vi "AlliGator Get Phasor Plot Parameters.vi"(8 "Error In":errorcluster) -> (0 "Error Out":errorcluster, 3 "Phasor Plot Parameters":T1={"Phasor Frequency"=0.0, "Decay Preprocessing Options & Parameters"={"Background Subtraction Parameters"={"Background Definition Range"={"Min Gate"=0.0, "Max Gate"=0.0}, "Baseline Subtraction Method"=enum."Mean", "Background Subtraction?"=FALSE, "Background File"=path "", "Background Constant"=0.0, "Background Scaling Factor"=1.0, "Background Pile-up Correction"=FALSE, "Background Pixel Well Capacity"=1}, "Decay Preprocessing Parameters"={"Background Subtraction"=FALSE, "Straighten Decay"=FALSE, "Reverse Gates"=FALSE, "1-Normalized Decay"=FALSE, "Smoothen Decay"=FALSE, "Smoothing Parameter"=0.0, "Shift Decay"=FALSE, "Decay Shift Parameters"={"Type"=enum."Default", "Shift"=0.0, "Threshold"=0.0, "Rotate"=FALSE}, "Extrapolate Decay"=FALSE, "Additional Points"=0, "Head Fraction"=0.0, "Pixel-Normalize Decay"=FALSE, "Use Periodicity"=FALSE, "Use Cursors"=FALSE, "Tail Fraction"=0.0, "Use Decay Pre-Processing"=TRUE, "Fold Decay"=FALSE, "# Folds"=1, "[0-1]-Normalized Decay"=FALSE}, "Preprocessing Steps Order"=[]}, "FLI Dataset Modified"=FALSE, "Source Image Settings"={"Low Count Pixels Rejection Options"={"Background Low Threshold Factor"=0.0, "Fixed Low Background Threshold"=0.0, "Reject Low Count Pixels"=FALSE, "Low Percentile"=0.0}, "High Count Pixels Rejection Options"={"Background High Threshold Factor"=0.0, "Fixed High Background Threshold"=20000.0, "Reject High Count Pixels"=FALSE, "High Percentile"=100.0}}, "Data Information"={"Gate Width"=0.0, "Gate Separation"=0.0, "Step (Gate Separation)"=0, "Laser Period"=0.0, "SYNC Period"=0.0, "Channel Name"=0, "Channel Arithmetic"=enum."None", "Pile-up Correction"=FALSE, "Pixel Well Capacity"=1, "Dataset Scaling Factor"=1.0}, "Phasor Plot"={"Phasor Plot Smoothing Options"={"Use Phasor Plot Smoothing"=FALSE, "Kernel Type"=enum."Uniform", "Bin"=1, "Algorithm"=enum."Rapid"}, "Phasor Plot Size"={"H"=0, "V"=0, "Margin"=0.0}, "Selected Image ROI(s)"=FALSE, "All Image ROIs"=FALSE, "Selected Source Image ROI"=0, "Source Image ROIs"=[]}} {"Phasor Plot"."Source Image ROIs"."ROI Descriptor"."Contours"."Type" items=["No Selection", "Point", "Line", "Rectangle", "Oval", "Polygon", "Freehand Region", "Annulus", "Unused2", "Unused3", "Broken Line", "Freehand Line", "Rotated Rectangle"]; "Phasor Plot"."Phasor Plot Smoothing Options"."Bin" min=1 step=2; "Data Information"."Dataset Scaling Factor" min=0.0; "Data Information"."Pixel Well Capacity" min=1 step=1; "Data Information"."Channel Name" items=["Gate"]; "Source Image Settings"."High Count Pixels Rejection Options"."High Percentile" min=0.0 max=100.0; "Source Image Settings"."Low Count Pixels Rejection Options"."Low Percentile" min=0.0 max=100.0; "Decay Preprocessing Options & Parameters"."Decay Preprocessing Parameters"."# Folds" min=1; "Decay Preprocessing Options & Parameters"."Background Subtraction Parameters"."Background Pixel Well Capacity" min=1 step=1; "Phasor Frequency" min=-2147483648.0 max=2147483647.0}, 4 "CPU (s)":dbl)   [LabVIEW 2021, in "AlliGator Phasor Plot.lvlib"]
doc: "Returns a structure with all the options needed to build the Phasor Plot image."
uses:
  AlliGator Phasor Plot.lvlib
  AlliGator Phasor Plot Parameters v2.ctl
  Decay Analysis/Decay Preprocessing/AlliGator Decay Preprocessing Options.ctl
  Decay Analysis/Decay Preprocessing/AlliGator Background Subtraction Parameters.ctl
  Decay Analysis/Decay Preprocessing/AlliGator Baseline Subtraction Method.ctl
  Decay Analysis/Decay Preprocessing/AlliGator Decay Preprocessing Parameters.ctl
  Graphs/XY Graph/XY Graph Plot Shift Parameters.ctl
  Graphs/XY Graph/XY Graph Plot Shift Method.ctl
  Settings/AlliGator Low Count Pixels Rejection Options.ctl
  Settings/AlliGator High Count Pixels Rejection Options.ctl
  Settings/AlliGator Gate Arithmetic.ctl
  AlliGator Phasor Plot Smoothing Options.ctl
  Arrays/Kernel Type.ctl
  Arrays/Smoothing Algorithm.ctl
  AlliGator Phasor Plot Size.ctl
  Image/Named ROI Description.ctl
  Settings/AlliGator Settings List.ctl
  Globals, Variables, Constants/AlliGator Variables List.ctl
  Variant/Variant to Data/Variant to I32.vi
  Variant/Variant to Data/Variant to Boolean.vi
  Settings/AlliGator Settings.lvlib
  Arrays/Arrays.lvlib
  Variant/Variant to Data/Variant to Data.lvlib
  Graphs/XY Graph/XY Graph Add-Ons.lvlib
  Decay Analysis/Decay Preprocessing/AlliGator Decay Preprocessing.lvlib
  Globals, Variables, Constants/AlliGator Globals, Variables & Constants.lvlib
  Image/Image.lvlib
  Time/Time.lvlib
panel:
  # "see the AlliGator License on the block diagram (Ctrl+E or Window:Show Block Diagram)"
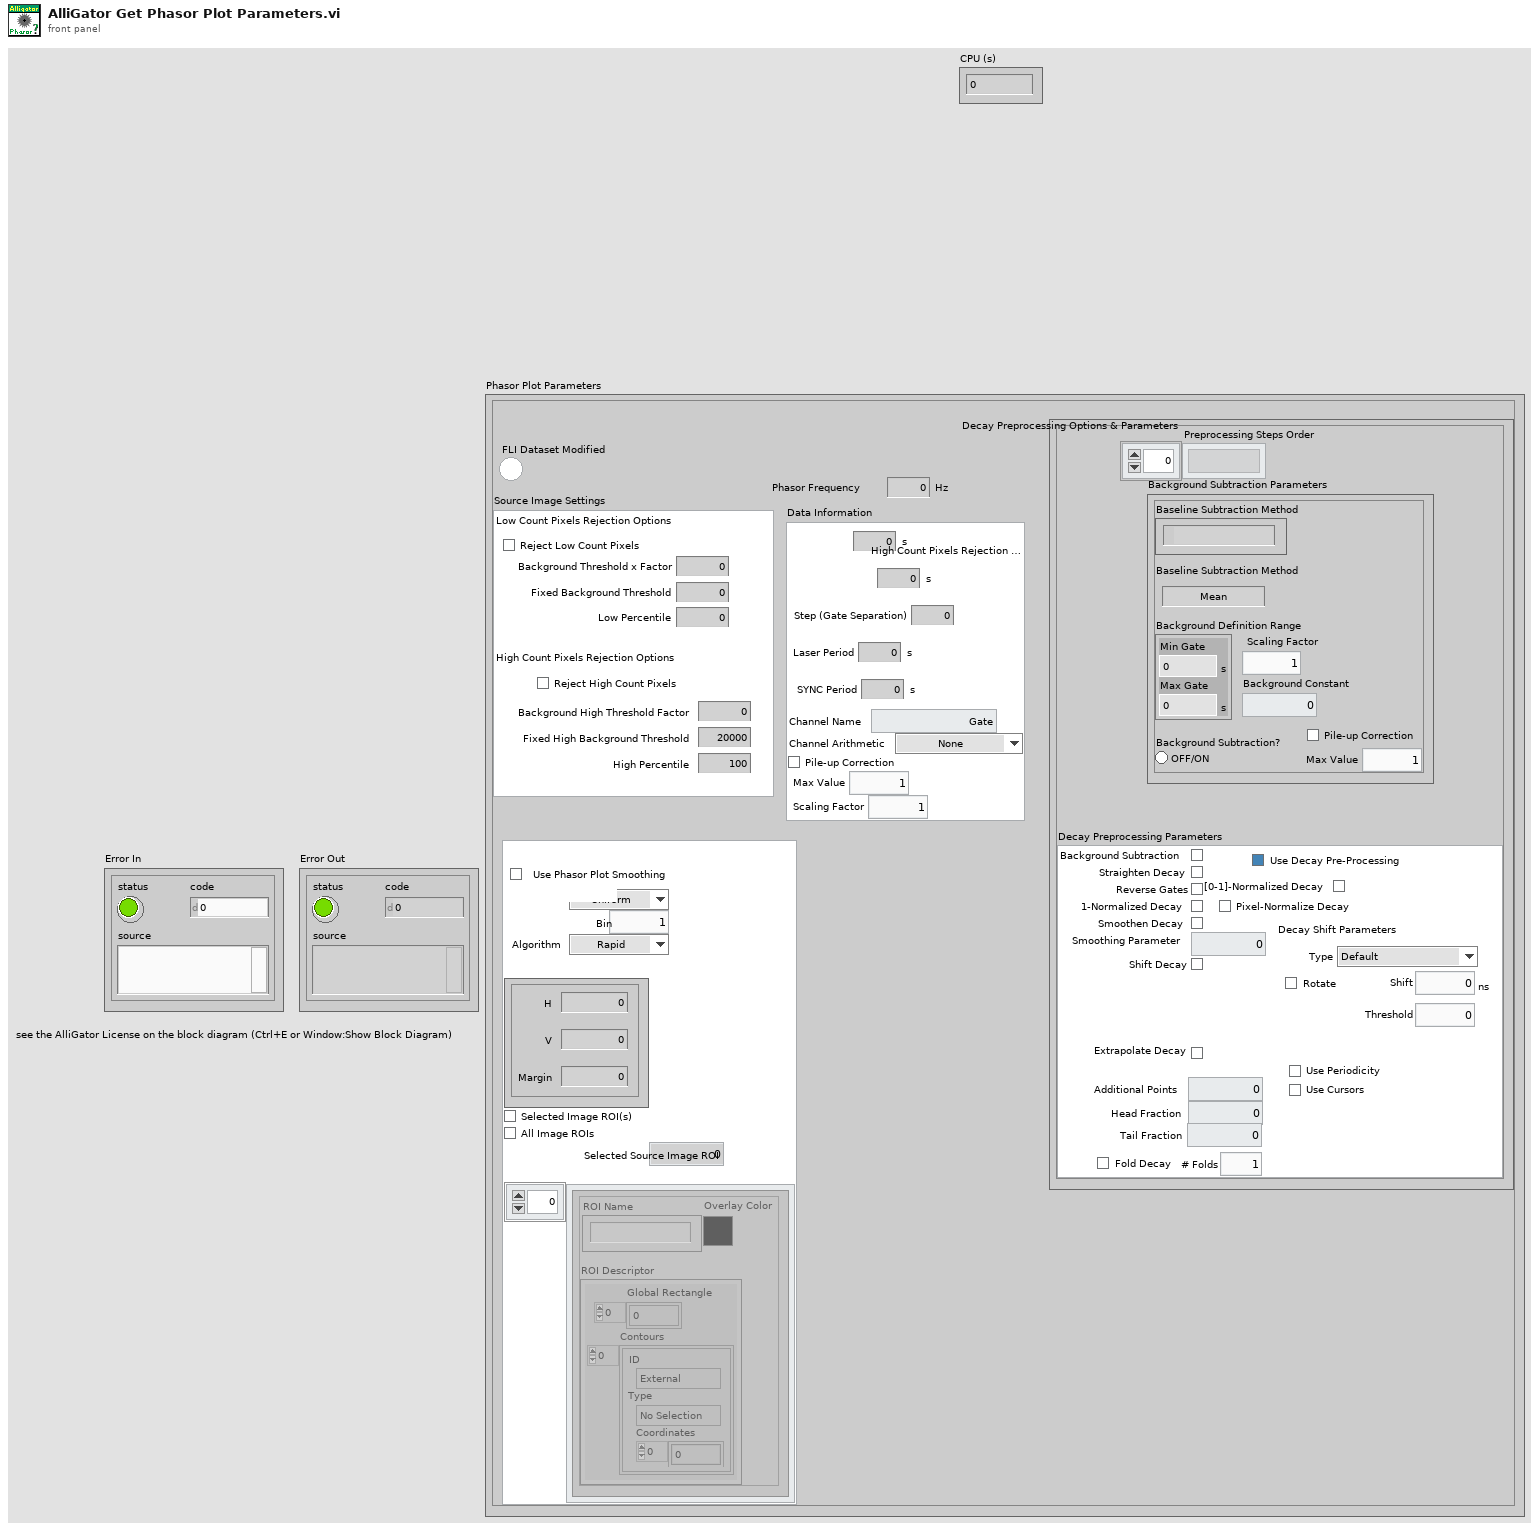
[diagram p1: front panel]
types:
  T1 = typedef "AlliGator Phasor Plot.lvlib/AlliGator Phasor Plot Parameters v2.ctl" = cluster{"Phasor Frequency":dbl[unit], "Decay Preprocessing Options & Parameters":T2, "FLI Dataset Modified":bool, "Source Image Settings":cluster{"Low Count Pixels Rejection Options":T8, "High Count Pixels Rejection Options":T9}, "Data Information":cluster{"Gate Width":dbl[unit], "Gate Separation":dbl[unit], "Step (Gate Separation)":i32, "Laser Period":dbl[unit], "SYNC Period":dbl[unit], "Channel Name":u16, "Channel Arithmetic":T10, "Pile-up Correction":bool, "Pixel Well Capacity":u32, "Dataset Scaling Factor":dbl}, "Phasor Plot":cluster{"Phasor Plot Smoothing Options":T11, "Phasor Plot Size":T14, "Selected Image ROI(s)":bool, "All Image ROIs":bool, "Selected Source Image ROI":i32, "Source Image ROIs":T15[]}}
  T2 = typedef "AlliGator Decay Preprocessing.lvlib/AlliGator Decay Preprocessing Options.ctl" = cluster{"Background Subtraction Parameters":T3, "Decay Preprocessing Parameters":T5, "Preprocessing Steps Order":string[]}
  T3 = typedef "AlliGator Decay Preprocessing.lvlib/AlliGator Background Subtraction Parameters.ctl" = cluster{"Background Definition Range":cluster{"Min Gate":dbl[unit], "Max Gate":dbl[unit]}, "Baseline Subtraction Method":T4, "Background Subtraction?":bool, "Background File":path, "Background Constant":dbl, "Background Scaling Factor":dbl, "Background Pile-up Correction":bool, "Background Pixel Well Capacity":u32}
  T4 = typedef "AlliGator Decay Preprocessing.lvlib/AlliGator Baseline Subtraction Method.ctl" = enum16{"Mean", "Min", "Square Gated Single-Exponential", "File", "Constant"}
  T5 = typedef "AlliGator Decay Preprocessing.lvlib/AlliGator Decay Preprocessing Parameters.ctl" = cluster{"Background Subtraction":bool, "Straighten Decay":bool, "Reverse Gates":bool, "1-Normalized Decay":bool, "Smoothen Decay":bool, "Smoothing Parameter":dbl, "Shift Decay":bool, "Decay Shift Parameters":T6, "Extrapolate Decay":bool, "Additional Points":u32, "Head Fraction":dbl, "Pixel-Normalize Decay":bool, "Use Periodicity":bool, "Use Cursors":bool, "Tail Fraction":dbl, "Use Decay Pre-Processing":bool, "Fold Decay":bool, "# Folds":u32, "[0-1]-Normalized Decay":bool}
  T6 = typedef "XY Graph Add-Ons.lvlib/XY Graph Plot Shift Parameters.ctl" = cluster{"Type":T7, "Shift":dbl[unit], "Threshold":dbl, "Rotate":bool}
  T7 = typedef "XY Graph Add-Ons.lvlib/XY Graph Plot Shift Method.ctl" = enum16{"Default", "CFD", "Threshold", "Cross-Correlation"}
  T8 = typedef "AlliGator Settings.lvlib/AlliGator Low Count Pixels Rejection Options.ctl" = cluster{"Background Low Threshold Factor":dbl, "Fixed Low Background Threshold":dbl, "Reject Low Count Pixels":bool, "Low Percentile":dbl}
  T9 = typedef "AlliGator Settings.lvlib/AlliGator High Count Pixels Rejection Options.ctl" = cluster{"Background High Threshold Factor":dbl, "Fixed High Background Threshold":dbl, "Reject High Count Pixels":bool, "High Percentile":dbl}
  T10 = typedef "AlliGator Settings.lvlib/AlliGator Gate Arithmetic.ctl" = enum16{"None", "INT-G2", "G2/INT*<INT>", "(1 - G2/INT)*<INT>"}
  T11 = typedef "AlliGator Phasor Plot.lvlib/AlliGator Phasor Plot Smoothing Options.ctl" = cluster{"Use Phasor Plot Smoothing":bool, "Kernel Type":T12, "Bin":i32, "Algorithm":T13}
  T12 = typedef "Arrays.lvlib/Kernel Type.ctl" = enum16{"Uniform", "Bilinear", "Gaussian"}
  T13 = typedef "Arrays.lvlib/Smoothing Algorithm.ctl" = enum16{"Rapid", "Thorough"}
  T14 = typedef "AlliGator Phasor Plot.lvlib/AlliGator Phasor Plot Size.ctl" = cluster{"H":i32, "V":i32, "Margin":dbl}
  T15 = typedef "Image.lvlib/Named ROI Description.ctl" = cluster{"ROI Descriptor":T16, "ROI Name":string, "Overlay Color":u32}
  T16 = typedef "ROI Descriptor" = cluster{"Global Rectangle":i32[], "Contours":cluster{"ID":enum32{"External", "Internal"}, "Type":u32, "Coordinates":i32[]}[]}
  T17 = typedef "AlliGator Settings.lvlib/AlliGator Settings List.ctl" = enum16{"GUI:Visible Settings Tab", "GUI:Last Run Version", "Source Image:Use Image Histogram for Contrast", "Source Image:Low Count Pixels Rejection Options", "Source Image:High Count Pixels Rejection Options", "Source Image:Use Image Brightness", "Source Image:Blend Overlay with Image Background", "Source Image:Use Fixed ROI Diameter", "Source Image:ROI Diameter", "Source Image:ROI Center Color", "Source Image:Peak Threshold", "Source Image:Intensity Threshold", "Source Image:Image Binning Options", "Source Image:Image Smoothing Options", "Source Image:Image Histogram Active", "Source Image:Invert Binary Mask", "Source Image:Hot Pixel Removal", "Source Image:Overlay Analyzed ROI Center", "Source Image:Auto-Adjust Contrast", "Source Image:Histogram Lower Percentile", "Source Image:Histogram Upper Percentile", "Source Image:Save Source Image", "Source Image:Scale Bar Options", "Source Image:Image Resolution (Pixel Size)", "Source Image:Flatfield Correction", "Source Image:Show Dead Left Columns Correction", "Source Image:Dead Left Columns Correction", "Source Image:Image Pre-Processing Operations Order", "Source Image:Overlay ROI Median", "Source Image:Median Overlay Color", "Data Information:Gate Width", "Data Information:Nanotime Gate Separation", "Data Information:Macrotime Gate Separation", "Data Information:Gate Step", "Data Information:# Gates", "Data Information:Gate Image Exposure", "Data Information:Gate Image Integration", "Data Information:Gates to Skip", "Data Information:Gates to Keep", "Data Information:Define Gates to", "Data Information:Channel Name", "Data Information:Available Channel Names", "Data Information:Channel Arithmetic", "Data Information:Background File Subtraction", "Data Information:Background File", "Data Information:Background Scaling Factor", "Data Information:Background Pile-up Correction", "Data Information:Background Pixel Well Capacity", "Data Information:Laser Period", "Data Information:SYNC Period", "Data Information:Pile-up Correction", "Data Information:Pixel Well Capacity", "Data Information:Dataset Scaling Factor", "Fluorescence Decay_Decay Pre-Processing:Reverse Gates", "Fluorescence Decay_Decay Pre-Processing:Verbose Decay Pre-Processing", "Fluorescence Decay_Decay Pre-Processing:Use Decay Pre-Processing", "Fluorescence Decay_Decay Pre-Processing:Background Subtraction", "Fluorescence Decay_Decay Pre-Processing:Background Definition Range", "Fluorescence Decay_Decay Pre-Processing:Baseline Subtraction Method", "Fluorescence Decay_Decay Pre-Processing:Decay Pre-Processing Operations Order", "Fluorescence Decay_Decay Pre-Processing:Smoothing Parameter", "Fluorescence Decay_Decay Pre-Processing:Shift Decay", "Fluorescence Decay_Decay Pre-Processing:Decay Shift Parameters", "Fluorescence Decay_Decay Pre-Processing:Fold Decay", "Fluorescence Decay_Decay Pre-Processing:# Folds", "Fluorescence Decay_Decay Pre-Processing:1-Normalize Decay", "Fluorescence Decay_Decay Pre-Processing:[0-1]-Normalize Decay", "Fluorescence Decay_Decay Pre-Processing:Smoothen Decay", "Fluorescence Decay_Decay Pre-Processing:Extrapolate Decay", "Fluorescence Decay_Decay Pre-Processing:Use Periodicity", "Fluorescence Decay_Decay Pre-Processing:Use Cursors", "Fluorescence Decay_Decay Pre-Processing:Tail Fraction", "Fluorescence Decay_Decay Pre-Processing:Head Fraction", "Fluorescence Decay_Decay Pre-Processing:Additional Points", "Fluorescence Decay_Decay Pre-Processing:Straighten Decay", "Fluorescence Decay_Decay Pre-Processing:Constant Background", "Fluorescence Decay_Decay Pre-Processing:Pixel-Normalize Decay", "Fluorescence Decay_Advanced Analysis:Extract IRF instead of Decay", "Fluorescence Decay_Advanced Analysis:IRF Extraction Options", "Fluorescence Decay_Advanced Analysis:IRF Optimization Options", "Fluorescence Decay_Advanced Analysis:Square Pulse Options", "Fluorescence Decay_Advanced Analysis:IRF Order", "Fluorescence Decay_Advanced Analysis:IRF Time Constants", "Fluorescence Decay_Advanced Analysis:Wavelet Analysis Options", "Fluorescence Decay_Advanced Analysis:Average Lifetime Options", "Fluorescence Decay_Fit Options:Fit Options", "Fluorescence Decay_Fit Options:Use Legacy Fitting Approach", "Fluorescence Decay_Fit Options:Use Data Information Laser Period", "Fluorescence Decay_Fit Parameters:Displayed Fit Parameters", "Fluorescence Decay_Fit Parameters:Fit Parameter Constraints", "Fluorescence Decay_Fit Parameters:Export Tabulated Results", "Fluorescence Decay_Fit Parameters:MLE Baseline Offset Type", "Fluorescence Decay_Fit Parameters:MLE Baseline Offset", "Fluorescence Decay_Fit Parameters:Guess Parameter Names", "Fluorescence Decay_Fit Parameters:Guess Parameter Values", "Fluorescence Decay_Fit Parameters:Guess Parameters Options", "Fluorescence Decay_Styles:Show Last Decay Only", "Fluorescence Decay_Styles:Decay Graph Color Array", "Fluorescence Decay:Decay Graph Active", "Fluorescence Decay Statistics:Min Peak Value", "Fluorescence Decay Statistics:Reject Low Decay Peak Pixels", "Fluorescence Decay Statistics:Reject High Decay Peak Pixels", "Fluorescence Decay Statistics:Max Peak Value", "Time Traces:Use File Timestamp", "Time Traces:Time Step", "Time Traces:Use Intensity Correction File", "Time Traces:Intensity Correction File", "Phasor Plot:Phasor Plot Smoothing Options", "Phasor Plot:Phasor Plot Size", "Phasor Plot:Phasor Plot Graphics Options", "Phasor Plot:Cumulative Phasor Plot", "Phasor Plot:Use Phasor Brightness", "Phasor Plot:Blend Overlay with Phasor Background", "Phasor Plot:Save Phasor Plot", "Phasor Plot:Show References", "Phasor Plot:Phasor Ratio Decay Range", "Phasor Plot:Exponential Fading", "Phasor Plot:Phasor Ratio Reference Colors", "Phasor Plot:Reference Radius", "Phasor Plot:Show Color Map Vertices", "Phasor Plot:Phasor Plot Active", "Phasor Plot:Phasor Ratio Color Map Type", "Phasor Plot:Phasor Ratio Color Map", "Phasor Plot:Phasor Ratio Display Range", "Phasor Plot:Selected Image ROI(s)", "Phasor Plot:All Image ROIs", "Phasor Plot:Selected Phasor Plot ROI(s)", "Phasor Plot:All Phasor Plot ROIs", "Phasor Plot:Phasor Ratio Color-Coded Quantity", "Phasor Plot:Store Phasor Harmonics", "Phasor Plot:Draw Reference Segment", "Phasor Plot:User-Defined Quantity", "Phasor Graph:Phasor Frequency", "Phasor Graph:Phasor Ratio Type", "Phasor Graph:Pixel-level Phasor Computation", "Phasor Graph:Save Phasor Graph", "Phasor Graph:Phasor Graph Active", "Phasor Graph:Phasor SDV Options", "Phasor Calibration:Use Backup Calibration if needed", "Phasor Graph:Define Shortest Lifetime as", "Phasor Calibration:Backup Calibration Type", "Phasor Calibration:Calibration Type", "Phasor Calibration:Calibration Lifetime", "Phasor Calibration:Calibration Map Algorithm", "Single-Exponential Phasor Locus (SEPL):Gate Parameters", "Single-Exponential Phasor Locus (SEPL):User-defined Gate", "Single-Exponential Phasor Locus (SEPL):User-defined IRF", "Single-Exponential Phasor Locus (SEPL):Phasor Parameters", "Single-Exponential Phasor Locus (SEPL):Decay & IRF Parameters", "Single-Exponential Phasor Locus (SEPL):Display Parameters", "Lifetime Analysis:Decay Analysis Parameters", "Lifetime Analysis:Lifetime Map Active", "Plugins:Python Settings", "Miscellaneous:Verbose Mode", "Miscellaneous:Beep after Script", "Miscellaneous:Saved Image File Format", "Miscellaneous:Exported Gate Image Settings", "Miscellaneous:Include Loading in Timing", "Miscellaneous:Verbose Settings Mode", "Miscellaneous:Histogram Options", "Miscellaneous:Beep on Error", "Miscellaneous:# Logical Processors Used", "Miscellaneous:ROI Description Max Characters", "Miscellaneous:Verbose Error Mode", "Miscellaneous:Transparent Mask Color"}
  T18 = typedef "AlliGator Globals, Variables & Constants.lvlib/AlliGator Variables List.ctl" = enum16{"---- GUI ----", "GUI:Initialization Status", "GUI:State Indicators Refnum", "GUI:Original AlliGator Menu Items", "GUI:Current Action Loop State", "GUI:Script in progress", "GUI:Playback", "GUI:Loop Playback", "GUI:Search ROI Used", "GUI:Search ROI", "Decay Graph Max Legend Size", "Intensity Graph Max Legend Size", "Decay Statistics Graph Max Legend Size", "Phasor Graph Max Legend Size", "Phasor Ratio Graph Max Legend Size", "Lifetime Graph Max Legend Size", "---- Files ----", "Files:Export Dataset Frames as Individual Files", "Files:Show Batch Export Help Balloons", "Files:Frames in Dataset", "Files:ptu File Frame Start Indices", "Files:Current Frame in Dataset", "Files:Current Frame Timestamp", "Files:Dataset Loaded", "Files:Dataset Metadata", "Files:Dataset Channel", "Files:Dataset Data Description", "Files:Background Dataset Metadata", "Files:Background Dataset Channel", "Files:Background Dataset Data Description", "Files:Background File Subtraction", "Files:Background File Path", "Files:Background File Pile-up Correction", "Files:Background File Pixel Well Capacity", "Files:Background File Scaling Factor", "Files:Current Dataset Load Settings", "Files:Dataset Path", "Files:ICCD-specific Information", "Files:Macrotime Gate Separation", "------ Python Plugins ------", "Python Plugins:Information", "Python Plugins:Python Session", "Python Plugins:Valid Python Session?", "---- Source Image ----", "Source Image:ROIs", "Source Image:Current ROI", "Source Image:ROI Event Refnum", "X_Source Image Display Range", "X_Source Image Palette Information", "X_Type of Displayed Image", "X_Time Gate Slider", "Source Image:Palette List", "Source Image:Scale", "Source Image:ROI Overlay Color", "Source Image:Overlay to Erase", "Source Image:Is Displayed Image Accumulated", "Source Image:White Light Image Modified", "Source Image:Mask Image Modified", "---- Image Profile Window ----", "Image Profile:Window Event Refnum", "Image Profile:IntensityType", "Image Profile:Intensity Average Type", "Image Profile:Intensity-weighted SDV", "Image Profile:Box Profile Type", "Image Profile:Window Open", "Image Profile:Plotted Fit Parameter", "------ Phasor Graph -------", "Phasor Graph:Show Line", "---- Phasor Plot ---", "Phasor Plot:Parameters Changed", "Phasor Plot:FLI Dataset Modified since last Calculation", "Phasor Harmonics Data", "Selected Phasor Harmonics", "Phasor Harmonic Manager Event Refnum", "Phasor Plot:ROIs", "Phasor Plot:Current ROI", "Phasor Plot:ROI Event Refnum", "Phasor Plot:Image Reference Points", "Phasor Plot:Computed", "Phasor Plot:Palette Information", "Phasor Plot:Palette List", "Phasor Plot:Phasor Ratio Palette Information", "Phasor Plot:Phasor Ratio Palette List", "Phasor Plot:Image Scale", "Phasor Plot:Image Overlay to Erase", "Phasor Plot:Image Elements to Update", "Phasor Plot:Current Calculation Parameters", "Phasor Plot:Current Calibration Options", "Phasor Plot:Reset Cumulated Phasor Plot", "Phasor Plot:Reference 1", "Phasor Plot:Lifetime Reference 1", "Phasor Plot:Reference 1 Frequency", "Phasor Plot:Reference 2", "Phasor Plot:Lifetime Reference 2", "Phasor Plot:Reference 2 Frequency", "---- Decay Analysis ----", "Number of Selected Decays to Fit", "LS Fit Results", "LAR Fit Results", "BS Fit Results", "Last Decay Max - Min", "Best Fit Parameters", "Best Fit Parameter Names", "Actual Size X", "Actual Size Y", "Binning X", "Binning Y", "Actual # Gates", "Dataset Number", "Gates to...", "Gates Skipped", "Gates to keep", "Gate Step", "Gate Separation", "Reversed Gates", "Pile-up Correction", "Pixel Well Capacity", "Background Subtracted", "Background Subtraction Method", "Background Definition Range", "Background File (deprecated)", "Number of Dataset Accumulated", "Array of Accumulated Dataset Paths", "Do Averaged Datasets", "Destination File Path", "Process Plot Target", "Use 1/D as Phasor Frequency", "---- Decay Fit Parameter Map -----", "Decay Fit Parameter Map:Palette Information", "Decay Fit Parameter Map:Palette List", "---- Parameter Map ----", "Parameter Map:Palette Information", "Parameter Map:Palette List", "------- Local Decay Window ---------", "Local Decay Graph Window:Event Refnum", "Local Decay Graph Window:Use normalized IRF for convolution", "----- Miscellaneous ----", "Misc:Skippable Dialog Windows Status"}
  T19 = cluster{"Min Gate":dbl[unit], "Max Gate":dbl[unit]}
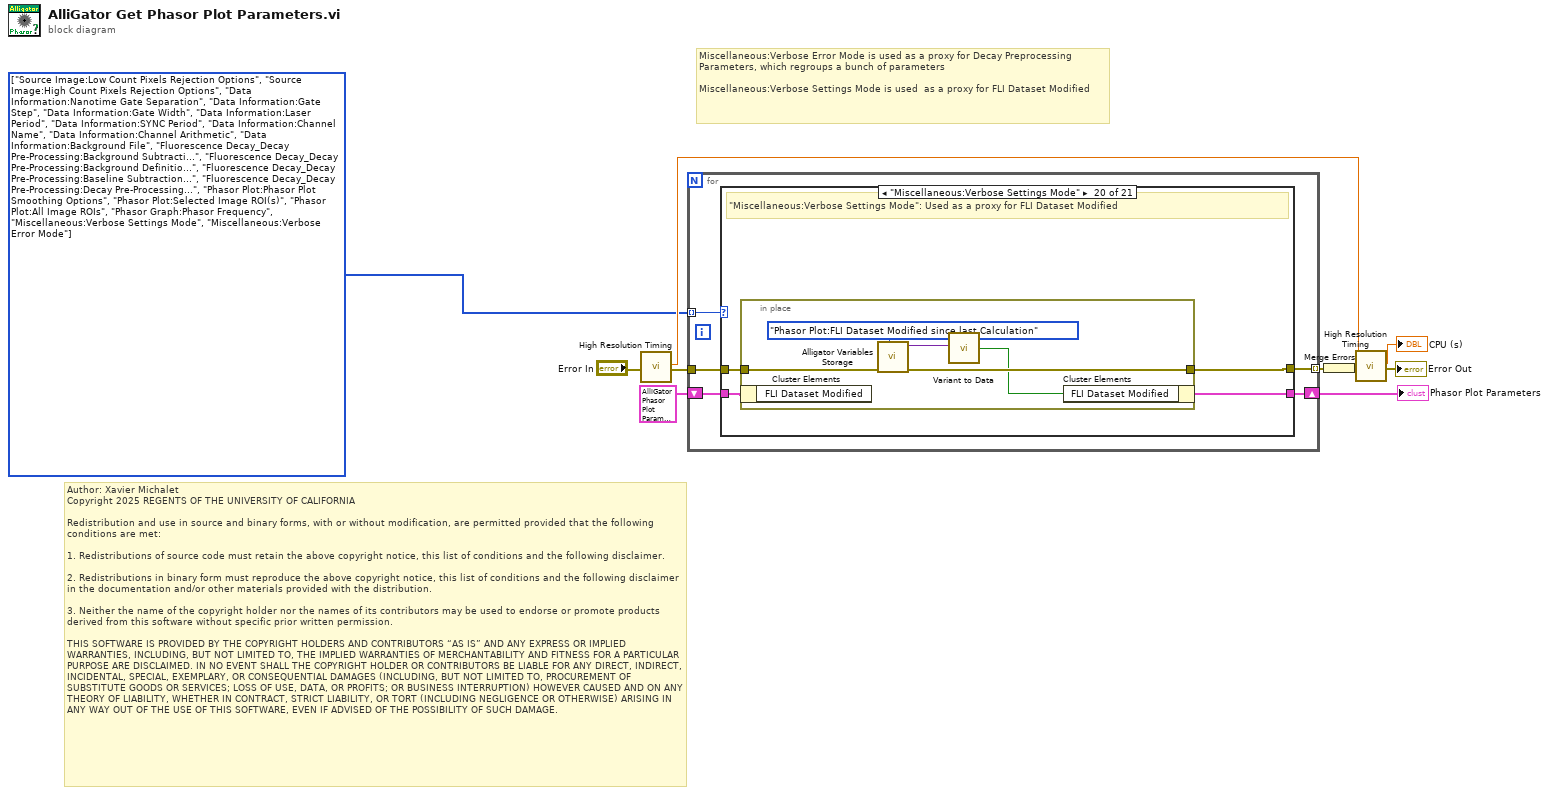
[diagram p0: block diagram]
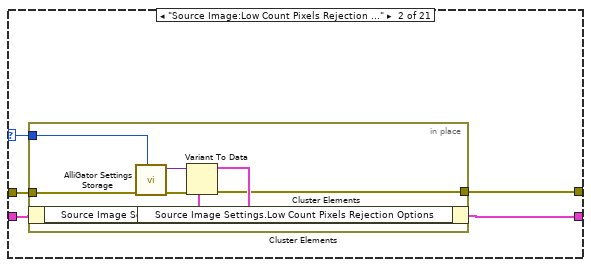
[diagram p3: hidden frame]
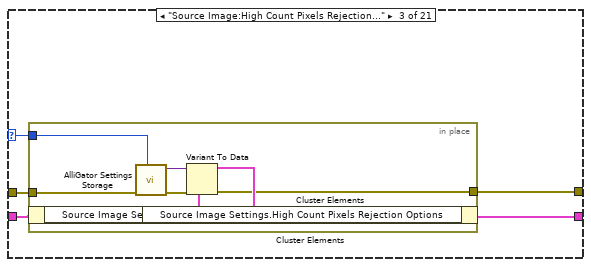
[diagram p4: hidden frame]
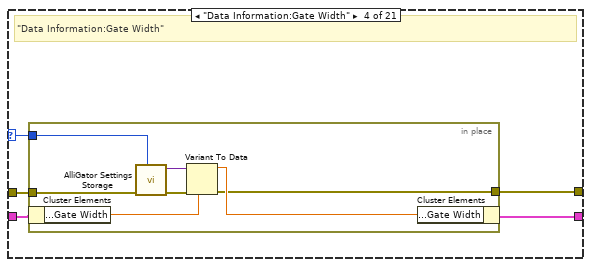
[diagram p5: hidden frame]
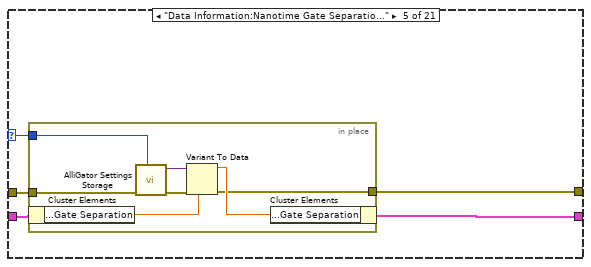
[diagram p6: hidden frame]
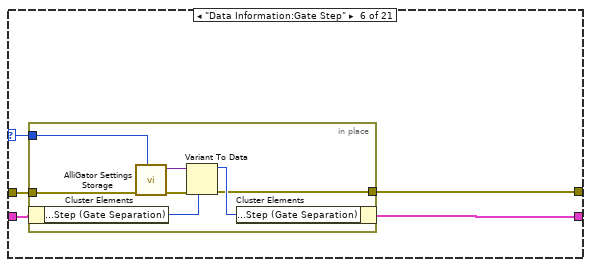
[diagram p7: hidden frame]
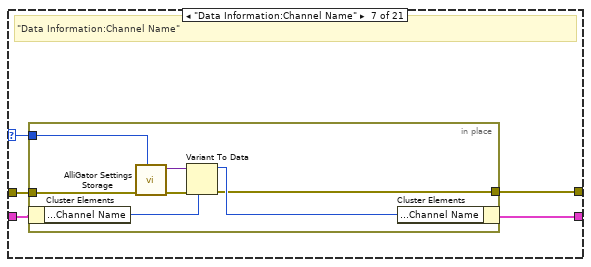
[diagram p8: hidden frame]
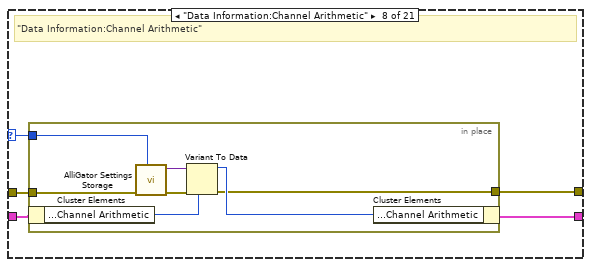
[diagram p9: hidden frame]
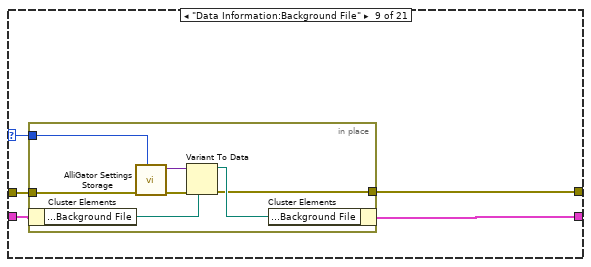
[diagram p10: hidden frame]
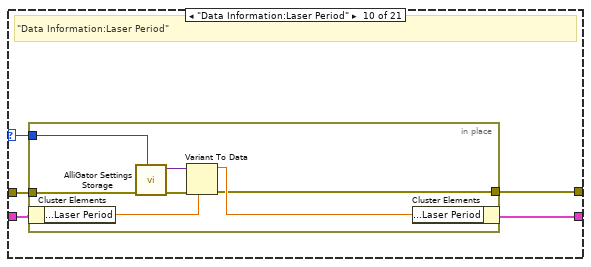
[diagram p11: hidden frame]
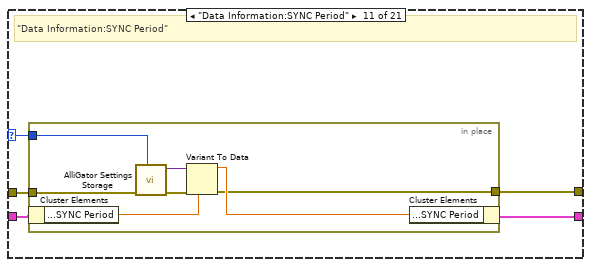
[diagram p12: hidden frame]
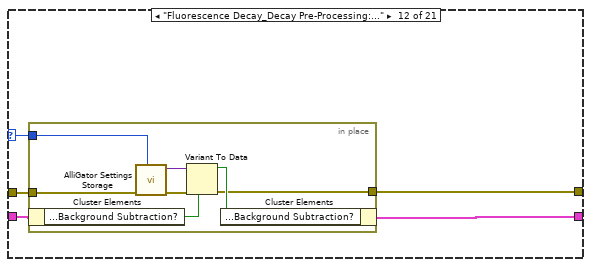
[diagram p13: hidden frame]
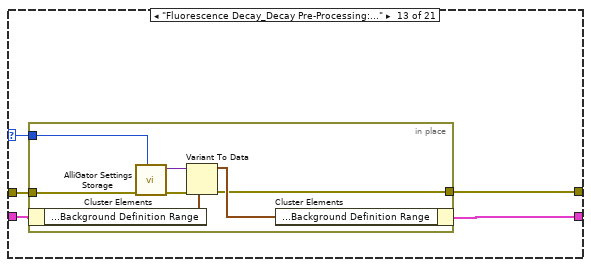
[diagram p14: hidden frame]
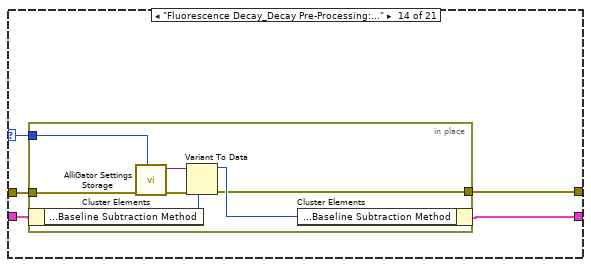
[diagram p15: hidden frame]
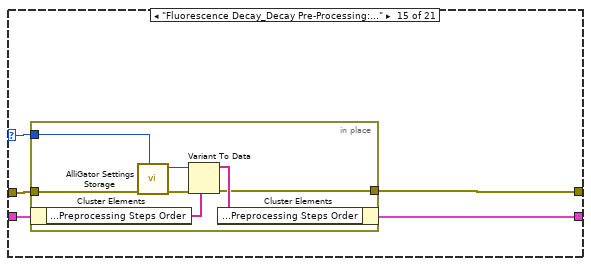
[diagram p16: hidden frame]
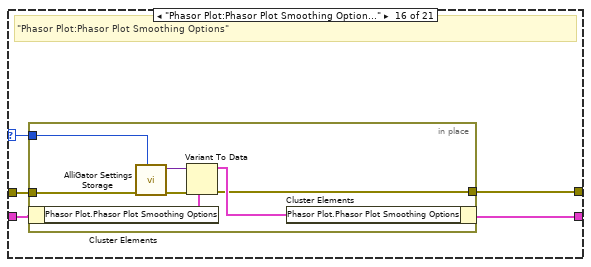
[diagram p17: hidden frame]
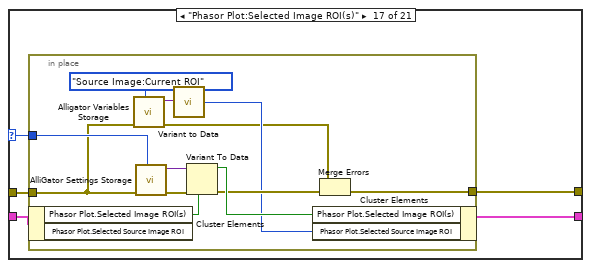
[diagram p18: hidden frame]
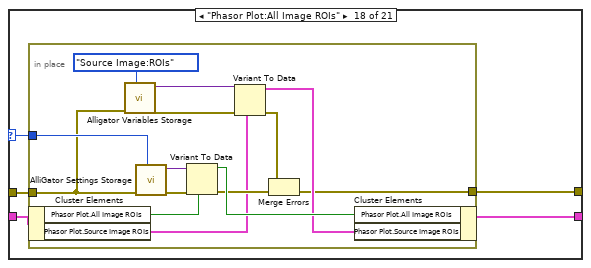
[diagram p19: hidden frame]
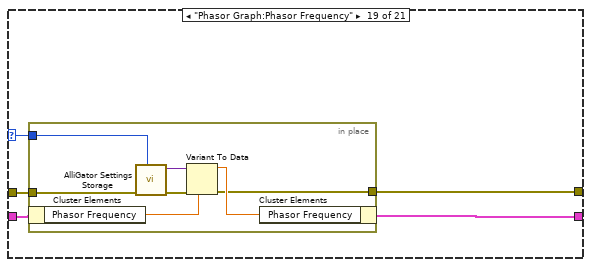
[diagram p20: hidden frame]
diagram:
  w1 = T17[] [enum."Source Image:Low Count Pixels Rejection Options", enum."Source Image:High Count Pixels Rejection Options", enum."Data Information:Nanotime Gate Separation", enum."Data Information:Gate Step", enum."Data Information:Gate Width", enum."Data Information:Laser Period", enum."Data Information:SYNC Period", enum."Data Information:Channel Name", enum."Data Information:Channel Arithmetic", enum."Data Information:Background File", enum."Fluorescence Decay_Decay Pre-Processing:Background Subtraction", enum."Fluorescence Decay_Decay Pre-Processing:Background Definition Range", enum."Fluorescence Decay_Decay Pre-Processing:Baseline Subtraction Method", enum."Fluorescence Decay_Decay Pre-Processing:Decay Pre-Processing Operations Order", enum."Phasor Plot:Phasor Plot Smoothing Options", enum."Phasor Plot:Selected Image ROI(s)", enum."Phasor Plot:All Image ROIs", enum."Phasor Graph:Phasor Frequency", enum."Miscellaneous:Verbose Settings Mode", enum."Miscellaneous:Verbose Error Mode"] items=["GUI:Visible Settings Tab", "GUI:Last Run Version", "Source Image:Use Image Histogram for Contrast", "Source Image:Low Count Pixels Rejection Options", "Source Image:High Count Pixels Rejection Options", "Source Image:Use Image Brightness", "Source Image:Blend Overlay with Image Background", "Source Image:Use Fixed ROI Diameter", "Source Image:ROI Diameter", "Source Image:ROI Center Color", "Source Image:Peak Threshold", "Source Image:Intensity Threshold", "Source Image:Image Binning Options", "Source Image:Image Smoothing Options", "Source Image:Image Histogram Active", "Source Image:Invert Binary Mask", "Source Image:Hot Pixel Removal", "Source Image:Overlay Analyzed ROI Center", "Source Image:Auto-Adjust Contrast", "Source Image:Histogram Lower Percentile", "Source Image:Histogram Upper Percentile", "Source Image:Save Source Image", "Source Image:Scale Bar Options", "Source Image:Image Resolution (Pixel Size)", "Source Image:Flatfield Correction", "Source Image:Show Dead Left Columns Correction", "Source Image:Dead Left Columns Correction", "Source Image:Image Pre-Processing Operations Order", "Source Image:Overlay ROI Median", "Source Image:Median Overlay Color", "Data Information:Gate Width", "Data Information:Nanotime Gate Separation", "Data Information:Macrotime Gate Separation", "Data Information:Gate Step", "Data Information:# Gates", "Data Information:Gate Image Exposure", "Data Information:Gate Image Integration", "Data Information:Gates to Skip", "Data Information:Gates to Keep", "Data Information:Define Gates to", "Data Information:Channel Name", "Data Information:Available Channel Names", "Data Information:Channel Arithmetic", "Data Information:Background File Subtraction", "Data Information:Background File", "Data Information:Background Scaling Factor", "Data Information:Background Pile-up Correction", "Data Information:Background Pixel Well Capacity", "Data Information:Laser Period", "Data Information:SYNC Period", "Data Information:Pile-up Correction", "Data Information:Pixel Well Capacity", "Data Information:Dataset Scaling Factor", "Fluorescence Decay_Decay Pre-Processing:Reverse Gates", "Fluorescence Decay_Decay Pre-Processing:Verbose Decay Pre-Processing", "Fluorescence Decay_Decay Pre-Processing:Use Decay Pre-Processing", "Fluorescence Decay_Decay Pre-Processing:Background Subtraction", "Fluorescence Decay_Decay Pre-Processing:Background Definition Range", "Fluorescence Decay_Decay Pre-Processing:Baseline Subtraction Method", "Fluorescence Decay_Decay Pre-Processing:Decay Pre-Processing Operations Order", "Fluorescence Decay_Decay Pre-Processing:Smoothing Parameter", "Fluorescence Decay_Decay Pre-Processing:Shift Decay", "Fluorescence Decay_Decay Pre-Processing:Decay Shift Parameters", "Fluorescence Decay_Decay Pre-Processing:Fold Decay", "Fluorescence Decay_Decay Pre-Processing:# Folds", "Fluorescence Decay_Decay Pre-Processing:1-Normalize Decay", "Fluorescence Decay_Decay Pre-Processing:[0-1]-Normalize Decay", "Fluorescence Decay_Decay Pre-Processing:Smoothen Decay", "Fluorescence Decay_Decay Pre-Processing:Extrapolate Decay", "Fluorescence Decay_Decay Pre-Processing:Use Periodicity", "Fluorescence Decay_Decay Pre-Processing:Use Cursors", "Fluorescence Decay_Decay Pre-Processing:Tail Fraction", "Fluorescence Decay_Decay Pre-Processing:Head Fraction", "Fluorescence Decay_Decay Pre-Processing:Additional Points", "Fluorescence Decay_Decay Pre-Processing:Straighten Decay", "Fluorescence Decay_Decay Pre-Processing:Constant Background", "Fluorescence Decay_Decay Pre-Processing:Pixel-Normalize Decay", "Fluorescence Decay_Advanced Analysis:Extract IRF instead of Decay", "Fluorescence Decay_Advanced Analysis:IRF Extraction Options", "Fluorescence Decay_Advanced Analysis:IRF Optimization Options", "Fluorescence Decay_Advanced Analysis:Square Pulse Options", "Fluorescence Decay_Advanced Analysis:IRF Order", "Fluorescence Decay_Advanced Analysis:IRF Time Constants", "Fluorescence Decay_Advanced Analysis:Wavelet Analysis Options", "Fluorescence Decay_Advanced Analysis:Average Lifetime Options", "Fluorescence Decay_Fit Options:Fit Options", "Fluorescence Decay_Fit Options:Use Legacy Fitting Approach", "Fluorescence Decay_Fit Options:Use Data Information Laser Period", "Fluorescence Decay_Fit Parameters:Displayed Fit Parameters", "Fluorescence Decay_Fit Parameters:Fit Parameter Constraints", "Fluorescence Decay_Fit Parameters:Export Tabulated Results", "Fluorescence Decay_Fit Parameters:MLE Baseline Offset Type", "Fluorescence Decay_Fit Parameters:MLE Baseline Offset", "Fluorescence Decay_Fit Parameters:Guess Parameter Names", "Fluorescence Decay_Fit Parameters:Guess Parameter Values", "Fluorescence Decay_Fit Parameters:Guess Parameters Options", "Fluorescence Decay_Styles:Show Last Decay Only", "Fluorescence Decay_Styles:Decay Graph Color Array", "Fluorescence Decay:Decay Graph Active", "Fluorescence Decay Statistics:Min Peak Value", "Fluorescence Decay Statistics:Reject Low Decay Peak Pixels", "Fluorescence Decay Statistics:Reject High Decay Peak Pixels", "Fluorescence Decay Statistics:Max Peak Value", "Time Traces:Use File Timestamp", "Time Traces:Time Step", "Time Traces:Use Intensity Correction File", "Time Traces:Intensity Correction File", "Phasor Plot:Phasor Plot Smoothing Options", "Phasor Plot:Phasor Plot Size", "Phasor Plot:Phasor Plot Graphics Options", "Phasor Plot:Cumulative Phasor Plot", "Phasor Plot:Use Phasor Brightness", "Phasor Plot:Blend Overlay with Phasor Background", "Phasor Plot:Save Phasor Plot", "Phasor Plot:Show References", "Phasor Plot:Phasor Ratio Decay Range", "Phasor Plot:Exponential Fading", "Phasor Plot:Phasor Ratio Reference Colors", "Phasor Plot:Reference Radius", "Phasor Plot:Show Color Map Vertices", "Phasor Plot:Phasor Plot Active", "Phasor Plot:Phasor Ratio Color Map Type", "Phasor Plot:Phasor Ratio Color Map", "Phasor Plot:Phasor Ratio Display Range", "Phasor Plot:Selected Image ROI(s)", "Phasor Plot:All Image ROIs", "Phasor Plot:Selected Phasor Plot ROI(s)", "Phasor Plot:All Phasor Plot ROIs", "Phasor Plot:Phasor Ratio Color-Coded Quantity", "Phasor Plot:Store Phasor Harmonics", "Phasor Plot:Draw Reference Segment", "Phasor Plot:User-Defined Quantity", "Phasor Graph:Phasor Frequency", "Phasor Graph:Phasor Ratio Type", "Phasor Graph:Pixel-level Phasor Computation", "Phasor Graph:Save Phasor Graph", "Phasor Graph:Phasor Graph Active", "Phasor Graph:Phasor SDV Options", "Phasor Calibration:Use Backup Calibration if needed", "Phasor Graph:Define Shortest Lifetime as", "Phasor Calibration:Backup Calibration Type", "Phasor Calibration:Calibration Type", "Phasor Calibration:Calibration Lifetime", "Phasor Calibration:Calibration Map Algorithm", "Single-Exponential Phasor Locus (SEPL):Gate Parameters", "Single-Exponential Phasor Locus (SEPL):User-defined Gate", "Single-Exponential Phasor Locus (SEPL):User-defined IRF", "Single-Exponential Phasor Locus (SEPL):Phasor Parameters", "Single-Exponential Phasor Locus (SEPL):Decay & IRF Parameters", "Single-Exponential Phasor Locus (SEPL):Display Parameters", "Lifetime Analysis:Decay Analysis Parameters", "Lifetime Analysis:Lifetime Map Active", "Plugins:Python Settings", "Miscellaneous:Verbose Mode", "Miscellaneous:Beep after Script", "Miscellaneous:Saved Image File Format", "Miscellaneous:Exported Gate Image Settings", "Miscellaneous:Include Loading in Timing", "Miscellaneous:Verbose Settings Mode", "Miscellaneous:Histogram Options", "Miscellaneous:Beep on Error", "Miscellaneous:# Logical Processors Used", "Miscellaneous:ROI Description Max Characters", "Miscellaneous:Verbose Error Mode", "Miscellaneous:Transparent Mask Color"] ("sorted array")
  # "Author: Xavier Michalet\nCopyright 2025 REGENTS OF THE UNIVERSITY OF CALIFORNIA\n\nRedistribution and use in source and binary forms, with or without modification, are permitted provided that the following conditions are met:\n\n1. Redistributions of source code must retain the above copyright notice, this list of conditions and the following disclaimer.\n\n2. Redistributions in binary form must reproduce the above copyright notice, this list of conditions and the following disclaimer in the documentation and/or other materials provided with the distribution.\n\n3. Neither the name of the copyright holder nor the names of its contributors may be used to endorse or promote products derived from this software without specific prior written permission.\n\nTHIS SOFTWARE IS PROVIDED BY THE COPYRIGHT HOLDERS AND CONTRIBUTORS “AS IS” AND ANY EXPRESS OR IMPLIED WARRANTIES, INCLUDING, BUT NOT LIMITED TO, THE IMPLIED WARRANTIES OF MERCHANTABILITY AND FITNESS FOR A PARTICULAR PURPOSE ARE DISCLAIMED. IN NO EVENT SHALL THE COPYRIGHT HOLDER OR CONTRIBUTORS BE LIABLE FOR ANY DIRECT, INDIRECT, INCIDENTAL, SPECIAL, EXEMPLARY, OR CONSEQUENTIAL DAMAGES (INCLUDING, BUT NOT LIMITED TO, PROCUREMENT OF SUBSTITUTE GOODS OR SERVICES; LOSS OF USE, DATA, OR PROFITS; OR BUSINESS INTERRUPTION) HOWEVER CAUSED AND ON ANY THEORY OF LIABILITY, WHETHER IN CONTRACT, STRICT LIABILITY, OR TORT (INCLUDING NEGLIGENCE OR OTHERWISE) ARISING IN ANY WAY OUT OF THE USE OF THIS SOFTWARE, EVEN IF ADVISED OF THE POSSIBILITY OF SUCH DAMAGE."
  # "Miscellaneous:Verbose Error Mode is used as a proxy for Decay Preprocessing Parameters, which regroups a bunch of parameters\n\nMiscellaneous:Verbose Settings Mode is used  as a proxy for FLI Dataset Modified"
  n1 = call "High Resolution Timing.vi"("Error In"="Error In") -> ("elapsed (relative) seconds"=w3:dbl, "Error Out"=w5:errorcluster)  [unwired: 16 in, 1 out]
  n2 = for {
    tunnel: w1 -> [w15] mode=indexing
    shift-right: [w13] -> w9
    shift-left: T1 {"Phasor Frequency"=0.0, "Decay Preprocessing Options & Parameters"={"Background Subtraction Parameters"={"Background Definition Range"={"Min Gate"=0.0, "Max Gate"=0.0}, "Baseline Subtraction Method"=enum."Mean", "Background Subtraction?"=FALSE, "Background File"=path "", "Background Constant"=0.0, "Background Scaling Factor"=1.0, "Background Pile-up Correction"=FALSE, "Background Pixel Well Capacity"=1}, "Decay Preprocessing Parameters"={"Background Subtraction"=FALSE, "Straighten Decay"=FALSE, "Reverse Gates"=FALSE, "1-Normalized Decay"=FALSE, "Smoothen Decay"=FALSE, "Smoothing Parameter"=0.0, "Shift Decay"=FALSE, "Decay Shift Parameters"={"Type"=enum."Default", "Shift"=0.0, "Threshold"=0.0, "Rotate"=FALSE}, "Extrapolate Decay"=FALSE, "Additional Points"=0, "Head Fraction"=0.0, "Pixel-Normalize Decay"=FALSE, "Use Periodicity"=FALSE, "Use Cursors"=FALSE, "Tail Fraction"=0.0, "Use Decay Pre-Processing"=TRUE, "Fold Decay"=FALSE, "# Folds"=1, "[0-1]-Normalized Decay"=FALSE}, "Preprocessing Steps Order"=[]}, "FLI Dataset Modified"=FALSE, "Source Image Settings"={"Low Count Pixels Rejection Options"={"Background Low Threshold Factor"=0.0, "Fixed Low Background Threshold"=0.0, "Reject Low Count Pixels"=FALSE, "Low Percentile"=0.0}, "High Count Pixels Rejection Options"={"Background High Threshold Factor"=0.0, "Fixed High Background Threshold"=20000.0, "Reject High Count Pixels"=FALSE, "High Percentile"=100.0}}, "Data Information"={"Gate Width"=0.0, "Gate Separation"=0.0, "Step (Gate Separation)"=0, "Laser Period"=0.0, "SYNC Period"=0.0, "Channel Name"=0, "Channel Arithmetic"=enum."None", "Pile-up Correction"=FALSE, "Pixel Well Capacity"=1, "Dataset Scaling Factor"=1.0}, "Phasor Plot"={"Phasor Plot Smoothing Options"={"Use Phasor Plot Smoothing"=FALSE, "Kernel Type"=enum."Uniform", "Bin"=1, "Algorithm"=enum."Rapid"}, "Phasor Plot Size"={"H"=0, "V"=0, "Margin"=0.0}, "Selected Image ROI(s)"=FALSE, "All Image ROIs"=FALSE, "Selected Source Image ROI"=0, "Source Image ROIs"=[]}} ("TG Phasor Plot Parameters") -> [w14]
    tunnel: w5 -> [w12]
    tunnel: [w11] -> w7 mode=indexing
    n3 = case shown="\"Miscellaneous:Verbose Settings Mode\"" w15 {
      selector: w15 -> [_ w22 w34 w46 w58 w70 w82 w94 w106 w118 w130 w142 w154 w166 w178 w190 w202 w219 w238 _ _]
      tunnel: w14 -> [w16 w21 w33 w45 w57 w69 w81 w93 w105 w117 w129 w141 w153 w165 w177 w189 w201 w218 w237 w249 w258]
      tunnel: [w16 w20 w32 w44 w56 w68 w80 w92 w104 w116 w128 w140 w152 w164 w176 w188 w200 w217 w236 w248 w257] -> w13
      tunnel: w12 -> [w17 w19 w31 w43 w55 w67 w79 w91 w103 w115 w127 w139 w151 w163 w175 w187 w199 w216 w235 w247 w256]
      tunnel: [w17 w18 w30 w42 w54 w66 w78 w90 w102 w114 w126 w138 w150 w162 w174 w186 w198 w215 w234 w246 w255] -> w11
      frame "GUI:Visible Settings Tab", Default {
      }
      frame "Source Image:Low Count Pixels Rejection Options" {
        n4 = in-place {
          in-place-border: w22 -> [w29]
          in-place-border: w19 -> [w24]
          in-place-border: [w23] -> w18
          n5 = in-place-cluster #1(w21) -> ("Source Image Settings.Low Count Pixels Rejection Options"=w26:T8)
          n6 = call "AlliGator Settings Storage.vi"("AlliGator Settings List"=w29, "Error In"=w24) -> ("Error Out"=w27:errorcluster, "Variant Data out"=w28:variant)  [unwired: 8 in]
          n7 = Variant To Data(error in=w27, type=w26, Variant=w28) -> (data=w25:T8, error out=w23:errorcluster)
          n8 = in-place-cluster #1("Source Image Settings.Low Count Pixels Rejection Options"=w25) -> (w20:T1)
        }
      }
      frame "Source Image:High Count Pixels Rejection Options" {
        n9 = in-place {
          in-place-border: w34 -> [w41]
          in-place-border: w31 -> [w36]
          in-place-border: [w35] -> w30
          n10 = in-place-cluster #2(w33) -> ("Source Image Settings.High Count Pixels Rejection Options"=w38:T9)
          n11 = call "AlliGator Settings Storage.vi"("AlliGator Settings List"=w41, "Error In"=w36) -> ("Error Out"=w39:errorcluster, "Variant Data out"=w40:variant)  [unwired: 8 in]
          n12 = Variant To Data(error in=w39, type=w38, Variant=w40) -> (data=w37:T9, error out=w35:errorcluster)
          n13 = in-place-cluster #2("Source Image Settings.High Count Pixels Rejection Options"=w37) -> (w32:T1)
        }
      }
      frame "Data Information:Gate Width" {
        # "\"Data Information:Gate Width\""
        n14 = in-place {
          in-place-border: w46 -> [w53]
          in-place-border: w43 -> [w48]
          in-place-border: [w47] -> w42
          n15 = in-place-cluster #3(w45) -> ("Data Information.Gate Width"=w50:dbl[unit])
          n16 = call "AlliGator Settings Storage.vi"("AlliGator Settings List"=w53, "Error In"=w48) -> ("Error Out"=w51:errorcluster, "Variant Data out"=w52:variant)  [unwired: 8 in]
          n17 = Variant To Data(error in=w51, type=w50, Variant=w52) -> (data=w49:dbl[unit], error out=w47:errorcluster)
          n18 = in-place-cluster #3("Data Information.Gate Width"=w49) -> (w44:T1)
        }
      }
      frame "Data Information:Nanotime Gate Separation" {
        n19 = in-place {
          in-place-border: w58 -> [w65]
          in-place-border: w55 -> [w60]
          in-place-border: [w59] -> w54
          n20 = in-place-cluster #4(w57) -> ("Data Information.Gate Separation"=w62:dbl[unit])
          n21 = call "AlliGator Settings Storage.vi"("AlliGator Settings List"=w65, "Error In"=w60) -> ("Error Out"=w63:errorcluster, "Variant Data out"=w64:variant)  [unwired: 8 in]
          n22 = Variant To Data(error in=w63, type=w62, Variant=w64) -> (data=w61:dbl[unit], error out=w59:errorcluster)
          n23 = in-place-cluster #4("Data Information.Gate Separation"=w61) -> (w56:T1)
        }
      }
      frame "Data Information:Gate Step" {
        n24 = in-place {
          in-place-border: w70 -> [w77]
          in-place-border: w67 -> [w72]
          in-place-border: [w71] -> w66
          n25 = in-place-cluster #5(w69) -> ("Data Information.Step (Gate Separation)"=w74:i32)
          n26 = call "AlliGator Settings Storage.vi"("AlliGator Settings List"=w77, "Error In"=w72) -> ("Error Out"=w75:errorcluster, "Variant Data out"=w76:variant)  [unwired: 8 in]
          n27 = Variant To Data(error in=w75, type=w74, Variant=w76) -> (data=w73:i32, error out=w71:errorcluster)
          n28 = in-place-cluster #5("Data Information.Step (Gate Separation)"=w73) -> (w68:T1)
        }
      }
      frame "Data Information:Channel Name" {
        # "\"Data Information:Channel Name\""
        n29 = in-place {
          in-place-border: w82 -> [w89]
          in-place-border: w79 -> [w84]
          in-place-border: [w83] -> w78
          n30 = in-place-cluster #6(w81) -> ("Data Information.Channel Name"=w86:u16)
          n31 = call "AlliGator Settings Storage.vi"("AlliGator Settings List"=w89, "Error In"=w84) -> ("Error Out"=w87:errorcluster, "Variant Data out"=w88:variant)  [unwired: 8 in]
          n32 = Variant To Data(error in=w87, type=w86, Variant=w88) -> (data=w85:u16, error out=w83:errorcluster)
          n33 = in-place-cluster #6("Data Information.Channel Name"=w85) -> (w80:T1)
        }
      }
      frame "Data Information:Channel Arithmetic" {
        # "\"Data Information:Channel Arithmetic\""
        n34 = in-place {
          in-place-border: w94 -> [w101]
          in-place-border: w91 -> [w96]
          in-place-border: [w95] -> w90
          n35 = in-place-cluster #7(w93) -> ("Data Information.Channel Arithmetic"=w98:T10)
          n36 = call "AlliGator Settings Storage.vi"("AlliGator Settings List"=w101, "Error In"=w96) -> ("Error Out"=w99:errorcluster, "Variant Data out"=w100:variant)  [unwired: 8 in]
          n37 = Variant To Data(error in=w99, type=w98, Variant=w100) -> (data=w97:T10, error out=w95:errorcluster)
          n38 = in-place-cluster #7("Data Information.Channel Arithmetic"=w97) -> (w92:T1)
        }
      }
      frame "Data Information:Background File" {
        n39 = in-place {
          in-place-border: w106 -> [w113]
          in-place-border: w103 -> [w108]
          in-place-border: [w107] -> w102
          n40 = in-place-cluster #8(w105) -> ("Decay Preprocessing Options & Parameters.Background Subtraction Parameters.Background File"=w110:path)
          n41 = call "AlliGator Settings Storage.vi"("AlliGator Settings List"=w113, "Error In"=w108) -> ("Error Out"=w111:errorcluster, "Variant Data out"=w112:variant)  [unwired: 8 in]
          n42 = Variant To Data(error in=w111, type=w110, Variant=w112) -> (data=w109:path, error out=w107:errorcluster)
          n43 = in-place-cluster #8("Decay Preprocessing Options & Parameters.Background Subtraction Parameters.Background File"=w109) -> (w104:T1)
        }
      }
      frame "Data Information:Laser Period" {
        # "\"Data Information:Laser Period\""
        n44 = in-place {
          in-place-border: w118 -> [w125]
          in-place-border: w115 -> [w120]
          in-place-border: [w119] -> w114
          n45 = in-place-cluster #9(w117) -> ("Data Information.Laser Period"=w122:dbl[unit])
          n46 = call "AlliGator Settings Storage.vi"("AlliGator Settings List"=w125, "Error In"=w120) -> ("Error Out"=w123:errorcluster, "Variant Data out"=w124:variant)  [unwired: 8 in]
          n47 = Variant To Data(error in=w123, type=w122, Variant=w124) -> (data=w121:dbl[unit], error out=w119:errorcluster)
          n48 = in-place-cluster #9("Data Information.Laser Period"=w121) -> (w116:T1)
        }
      }
      frame "Data Information:SYNC Period" {
        # "\"Data Information:SYNC Period\""
        n49 = in-place {
          in-place-border: w130 -> [w137]
          in-place-border: w127 -> [w132]
          in-place-border: [w131] -> w126
          n50 = in-place-cluster #10(w129) -> ("Data Information.SYNC Period"=w134:dbl[unit])
          n51 = call "AlliGator Settings Storage.vi"("AlliGator Settings List"=w137, "Error In"=w132) -> ("Error Out"=w135:errorcluster, "Variant Data out"=w136:variant)  [unwired: 8 in]
          n52 = Variant To Data(error in=w135, type=w134, Variant=w136) -> (data=w133:dbl[unit], error out=w131:errorcluster)
          n53 = in-place-cluster #10("Data Information.SYNC Period"=w133) -> (w128:T1)
        }
      }
      frame "Fluorescence Decay_Decay Pre-Processing:Background Subtraction" {
        n54 = in-place {
          in-place-border: w142 -> [w149]
          in-place-border: w139 -> [w144]
          in-place-border: [w143] -> w138
          n55 = in-place-cluster #11(w141) -> ("Decay Preprocessing Options & Parameters.Background Subtraction Parameters.Background Subtraction?"=w146:bool)
          n56 = call "AlliGator Settings Storage.vi"("AlliGator Settings List"=w149, "Error In"=w144) -> ("Error Out"=w147:errorcluster, "Variant Data out"=w148:variant)  [unwired: 8 in]
          n57 = Variant To Data(error in=w147, type=w146, Variant=w148) -> (data=w145:bool, error out=w143:errorcluster)
          n58 = in-place-cluster #11("Decay Preprocessing Options & Parameters.Background Subtraction Parameters.Background Subtraction?"=w145) -> (w140:T1)
        }
      }
      frame "Fluorescence Decay_Decay Pre-Processing:Background Definition Range" {
        n59 = in-place {
          in-place-border: w154 -> [w161]
          in-place-border: w151 -> [w156]
          in-place-border: [w155] -> w150
          n60 = in-place-cluster #12(w153) -> ("Decay Preprocessing Options & Parameters.Background Subtraction Parameters.Background Definition Range"=w158:T19)
          n61 = call "AlliGator Settings Storage.vi"("AlliGator Settings List"=w161, "Error In"=w156) -> ("Error Out"=w159:errorcluster, "Variant Data out"=w160:variant)  [unwired: 8 in]
          n62 = Variant To Data(error in=w159, type=w158, Variant=w160) -> (data=w157:T19, error out=w155:errorcluster)
          n63 = in-place-cluster #12("Decay Preprocessing Options & Parameters.Background Subtraction Parameters.Background Definition Range"=w157) -> (w152:T1)
        }
      }
      frame "Fluorescence Decay_Decay Pre-Processing:Baseline Subtraction Method" {
        n64 = in-place {
          in-place-border: w166 -> [w173]
          in-place-border: w163 -> [w168]
          in-place-border: [w167] -> w162
          n65 = in-place-cluster #13(w165) -> ("Decay Preprocessing Options & Parameters.Background Subtraction Parameters.Baseline Subtraction Method"=w170:T4)
          n66 = call "AlliGator Settings Storage.vi"("AlliGator Settings List"=w173, "Error In"=w168) -> ("Error Out"=w171:errorcluster, "Variant Data out"=w172:variant)  [unwired: 8 in]
          n67 = Variant To Data(error in=w171, type=w170, Variant=w172) -> (data=w169:T4, error out=w167:errorcluster)
          n68 = in-place-cluster #13("Decay Preprocessing Options & Parameters.Background Subtraction Parameters.Baseline Subtraction Method"=w169) -> (w164:T1)
        }
      }
      frame "Fluorescence Decay_Decay Pre-Processing:Decay Pre-Processing Operations Order" {
        n69 = in-place {
          in-place-border: w178 -> [w185]
          in-place-border: w175 -> [w180]
          in-place-border: [w179] -> w174
          n70 = in-place-cluster #14(w177) -> ("Decay Preprocessing Options & Parameters.Preprocessing Steps Order"=w182:string[])
          n71 = call "AlliGator Settings Storage.vi"("AlliGator Settings List"=w185, "Error In"=w180) -> ("Error Out"=w183:errorcluster, "Variant Data out"=w184:variant)  [unwired: 8 in]
          n72 = Variant To Data(error in=w183, type=w182, Variant=w184) -> (data=w181:string[], error out=w179:errorcluster)
          n73 = in-place-cluster #14("Decay Preprocessing Options & Parameters.Preprocessing Steps Order"=w181) -> (w176:T1)
        }
      }
      frame "Phasor Plot:Phasor Plot Smoothing Options" {
        # "\"Phasor Plot:Phasor Plot Smoothing Options\""
        n74 = in-place {
          in-place-border: w190 -> [w197]
          in-place-border: w187 -> [w192]
          in-place-border: [w191] -> w186
          n75 = in-place-cluster #15(w189) -> ("Phasor Plot.Phasor Plot Smoothing Options"=w194:T11)
          n76 = call "AlliGator Settings Storage.vi"("AlliGator Settings List"=w197, "Error In"=w192) -> ("Error Out"=w195:errorcluster, "Variant Data out"=w196:variant)  [unwired: 8 in]
          n77 = Variant To Data(error in=w195, type=w194, Variant=w196) -> (data=w193:T11, error out=w191:errorcluster)
          n78 = in-place-cluster #15("Phasor Plot.Phasor Plot Smoothing Options"=w193) -> (w188:T1)
        }
      }
      frame "Phasor Plot:Selected Image ROI(s)" {
        n79 = in-place {
          in-place-border: w202 -> [w214]
          in-place-border: w199 -> [w208]
          in-place-border: [w204] -> w198
          n80 = in-place-cluster #16(w201) -> ("Phasor Plot.Selected Image ROI(s)"=w211:bool)  [unwired: 1 out]
          n81 = call "Alligator Variables Storage.vi"("AlliGator Variable"=AlliGator_Variables_List."Source Image:Current ROI" ("Alligator Variable"), "Error In"=w208) -> ("Error Out"=w203:errorcluster, "Data out"=w206:variant)  [unwired: 7 in, 1 out]
          n82 = call "AlliGator Settings Storage.vi"("AlliGator Settings List"=w214, "Error In"=w208) -> ("Error Out"=w212:errorcluster, "Variant Data out"=w213:variant)  [unwired: 8 in]
          n83 = call-poly "Variant to Data.vi"("Variant"=w206) -> ("Value"=w205:i32)  [unwired: 8 in]
          n84 = Variant To Data(error in=w212, type=w211, Variant=w213) -> (data=w210:bool, error out=w209:errorcluster)
          n85 = in-place-cluster #16("Phasor Plot.Selected Image ROI(s)"=w210, "Phasor Plot.Selected Source Image ROI"=w205) -> (w200:T1)
          n86 = Merge Errors(w203, w209) -> (w204:errorcluster)
        }
      }
      frame "Phasor Plot:All Image ROIs" {
        n87 = in-place {
          in-place-border: w219 -> [w233]
          in-place-border: w216 -> [w226]
          in-place-border: [w222] -> w215
          n88 = in-place-cluster #17(w218) -> ("Phasor Plot.All Image ROIs"=w230:bool, "Phasor Plot.Source Image ROIs"=w225:T15[])
          n89 = call "Alligator Variables Storage.vi"("AlliGator Variable"=AlliGator_Variables_List."Source Image:ROIs" ("Alligator Variable"), "Error In"=w226) -> ("Error Out"=w223:errorcluster, "Data out"=w227:variant)  [unwired: 7 in, 1 out]
          n90 = call "AlliGator Settings Storage.vi"("AlliGator Settings List"=w233, "Error In"=w226) -> ("Error Out"=w231:errorcluster, "Variant Data out"=w232:variant)  [unwired: 8 in]
          n91 = Variant To Data(error in=w231, type=w230, Variant=w232) -> (data=w229:bool, error out=w228:errorcluster)
          n92 = Variant To Data(error in=w223, type=w225, Variant=w227) -> (data=w224:T15[], error out=w221:errorcluster)
          n93 = Merge Errors(w221, w228) -> (w222:errorcluster)
          n94 = in-place-cluster #17("Phasor Plot.All Image ROIs"=w229, "Phasor Plot.Source Image ROIs"=w224) -> (w217:T1)
        }
      }
      frame "Phasor Graph:Phasor Frequency" {
        n95 = in-place {
          in-place-border: w238 -> [w245]
          in-place-border: w235 -> [w240]
          in-place-border: [w239] -> w234
          n96 = in-place-cluster #18(w237) -> ("Phasor Frequency"=w242:dbl[unit])
          n97 = call "AlliGator Settings Storage.vi"("AlliGator Settings List"=w245, "Error In"=w240) -> ("Error Out"=w243:errorcluster, "Variant Data out"=w244:variant)  [unwired: 8 in]
          n98 = Variant To Data(error in=w243, type=w242, Variant=w244) -> (data=w241:dbl[unit], error out=w239:errorcluster)
          n99 = in-place-cluster #18("Phasor Frequency"=w241) -> (w236:T1)
        }
      }
      frame "Miscellaneous:Verbose Settings Mode" {
        # "\"Miscellaneous:Verbose Settings Mode\": Used as a proxy for FLI Dataset Modified"
        n100 = in-place {
          in-place-border: w247 -> [w254]
          in-place-border: [w253] -> w246
          n101 = in-place-cluster #19(w249) -> ()  [unwired: 1 out]
          n102 = call "Alligator Variables Storage.vi"("AlliGator Variable"=AlliGator_Variables_List."Phasor Plot:FLI Dataset Modified since last Calculation" ("Alligator Variable"), "Error In"=w254) -> ("Error Out"=w253:errorcluster, "Data out"=w251:variant)  [unwired: 7 in, 1 out]
          n103 = call-poly "Variant to Data.vi"("Variant"=w251) -> ("Value"=w250:bool)  [unwired: 8 in]
          n104 = in-place-cluster #19("FLI Dataset Modified"=w250) -> (w248:T1)
        }
      }
      frame "Miscellaneous:Verbose Error Mode" {
        # "\"Miscellaneous:Verbose Error Mode\": Used as a proxy for Decay Preprocessing Parameters"
        n105 = in-place {
          in-place-border: w256 -> [w261]
          in-place-border: [w260] -> w255
          n106 = in-place-cluster #20(w258) -> ()  [unwired: 1 out]
          n107 = call "AlliGator Get-Set Decay Preprocessing Options & Parameters.vi"("Get (F)/Set"=FALSE, "error in (no error)"=w261) -> ("error out"=w260:errorcluster, "Decay Preprocessing Options & Parameters out"=w263:T2)  [unwired: 8 in]
          n108 = Unbundle By Name(w263) -> ("Decay Preprocessing Parameters"=w262:T5)
          n109 = in-place-cluster #20("Decay Preprocessing Options & Parameters.Decay Preprocessing Parameters"=w262) -> (w257:T1)
        }
      }
    }
  }
  "Phasor Plot Parameters" <- w9
  n110 = Merge Errors(w7) -> (w6:errorcluster)
  n111 = call "High Resolution Timing.vi"("relative seconds (NaN)"=w3, "Error In"=w6) -> ("elapsed (relative) seconds"=→"CPU (s)":dbl, "Error Out"=→"Error Out":errorcluster)  [unwired: 15 in, 1 out]
